vi "Close.vi"(8 "error in":errorcluster, 11 "Server in":refnum<class "Server.lvclass">) -> (0 "error out":errorcluster, 3 "Server out":refnum<class "Server.lvclass">)   [LabVIEW 2020, in "Server.lvlib" / "Server.lvclass"]
uses:
  Server.lvclass
  Server.lvclass/Server.ctl
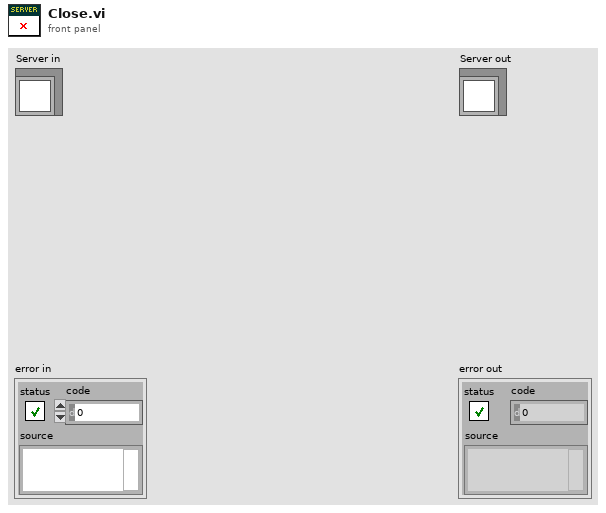
[diagram p1: front panel]
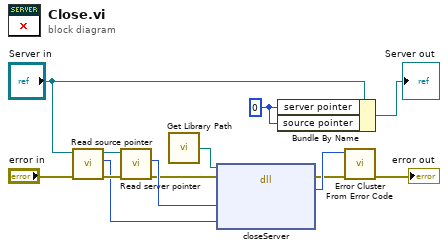
[diagram p0: block diagram]
diagram:
  w8 = i64 0
  n1 = call "Read source pointer.vi"("error in (no error)"="error in", "Server in"="Server in") -> ("error out"=w5:errorcluster, "source pointer"=w3:i64, "Server out"=w2:refnum<class "Server.lvclass">)  [unwired: 7 in]
  n2 = call "Read server pointer.vi"("error in (no error)"=w5, "Server in"=w2) -> ("error out"=w6:errorcluster, "server pointer"=w7:i64)  [unwired: 7 in, 1 out]
  n3 = call "Get Library Path.vi"() -> ("Path"=w9:path)  [unwired: 1 in]
  n4 = dll-call lib="?" fn="closeServer"(path in=w9, error in=w6, "server"=w7, "source"=w3) -> (error out=w10:errorcluster, "ret code"=w11:i32)  [unwired: 3 in, 1 out]
  n5 = Bundle By Name(cluster="Server in", "server pointer"=w8, "source pointer"=w8) -> (→"Server out":refnum<class "Server.lvclass">)
  n6 = call <vilib>:"Error Cluster From Error Code.vi"("error in (no error)"=w10, "error code (0)"=w11) -> ("error out"=→"error out":errorcluster)  [unwired: 7 in]
